vi "Hit Splitter.vi"(8 "error in (no error)":errorcluster, 10 "Coords":T2, 11 "IContainer in":refnum<class "IContainer.lvclass">) -> (0 "error out":errorcluster, 1 "Hit?":bool, 2 "Limits":cluster{"Left":i16, "Right":i16}, 3 "IContainer out":refnum<class "IContainer.lvclass">, 4 "Slider":T1={"Left"=0.0, "Top"=0.0, "Right"=1.0, "Bottom"=0.0}, 5 "vertical?":bool, 6 "Position":i16)   [LabVIEW 2021, in "IContainer.lvclass"]
doc: "Copyright 2018, Wiebe Walstra, wiebe@carya.nl."
uses:
  IContainer.lvclass
  <vilib>/Utility/miscctls.llb/LVPoint32TypeDef.ctl
  IContainer.lvclass/IContainer.ctl
  IObject.lvclass
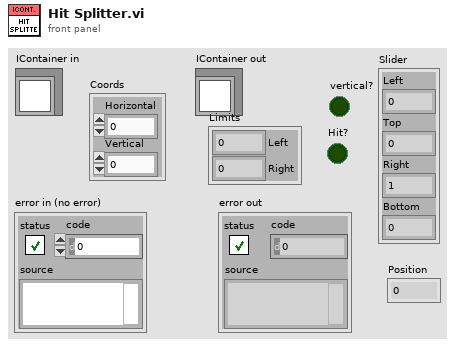
[diagram p1: front panel]
types:
  T1 = cluster{"Left":dbl, "Top":dbl, "Right":dbl, "Bottom":dbl}
  T2 = typedef "LVPoint32TypeDef.ctl" = cluster{"Horizontal":i32, "Vertical":i32}
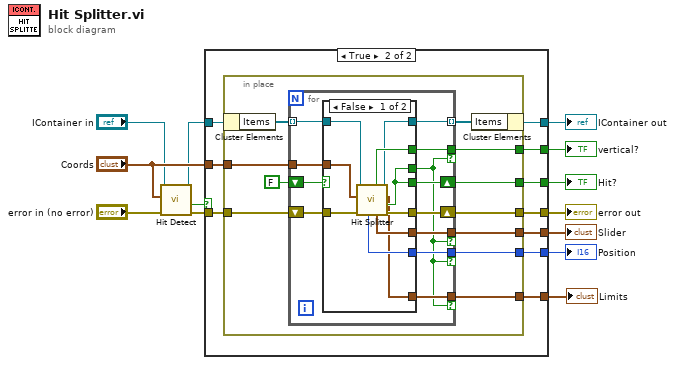
[diagram p0: block diagram]
diagram:
  n1 = call-dynamic "Hit Detect.vi"("error in (no error)"="error in (no error)", "Coords"="Coords", "IContainer in"="IContainer in") -> ("error out"=w8:errorcluster, "Hit?"=w3:bool, "IContainer out"=w1:refnum<class "IContainer.lvclass">)  [unwired: 5 in, 1 out]
  n2 = case shown="True" w3 {
    tunnel: [w15 w25] -> w13
    tunnel: [_ w24] -> w12
    tunnel: [_ w23] -> w11
    tunnel: [_ w22] -> w9
    tunnel: w8 -> [w15 w21]
    tunnel: w1 -> [w14 w18]
    tunnel: "Coords" -> [_ w20]
    tunnel: [w14 w17] -> w7
    tunnel: [_ w19] -> w6
    tunnel: [_ w16] -> w5
    frame False {
    }
    frame True {
      n3 = in-place {
        in-place-border: [w36] -> w25
        in-place-border: [w35] -> w24
        in-place-border: [w34] -> w23
        in-place-border: [w33] -> w22
        in-place-border: w21 -> [w32]
        in-place-border: w20 -> [w31]
        in-place-border: [w30] -> w19
        in-place-border: [w26] -> w16
        n4 = in-place-cluster #1(w18) -> ("Items"=w29:refnum<class "IObject.lvclass">[])
        n5 = for {
          tunnel: [w43] -> w34 if=w37
          tunnel: w31 -> [w46]
          shift-right: [w48] -> w36
          shift-left: w32 -> [w47]
          tunnel: [w45] -> w33 if=w37
          tunnel: [w44] -> w30 if=w37
          tunnel: w29 -> [w42] mode=indexing
          tunnel: [w41] -> w28 mode=indexing
          shift-right: [w39] -> w35
          shift-left: FALSE ("Hit?") -> [w40]
          tunnel: [w38] -> w26 if=w37
          n6 = case shown="False" w40 {
            selector: w40 -> [_ w60]
            tunnel: [w58 w59] -> w48
            tunnel: w47 -> [w57 w59]
            tunnel: w46 -> [w56 _]
            tunnel: [w55 _] -> w45
            tunnel: [w54 _] -> w44
            tunnel: [w53 _] -> w43
            tunnel: w42 -> [w52 w61]
            tunnel: [w51 w61] -> w41
            tunnel: [w50 w60] -> w39
            tunnel: [w50 _] -> w37
            tunnel: [w49 _] -> w38
            frame False {
              n7 = call-dynamic "Hit Splitter.vi"("error in (no error)"=w57, "Point32"=w56, "IObject in"=w52) -> ("error out"=w58:errorcluster, "Hit?"=w50:bool, "Limits"=w49:cluster{"Left":i16, "Right":i16}, "IObject out"=w51:refnum<class "IObject.lvclass">, "Slider"=w53:T1, "vertical?"=w55:bool, "Position"=w54:i16)  [unwired: 2 in]
            }
            frame True {
            }
          }
        }
        n8 = in-place-cluster #1("Items"=w28) -> (w17:refnum<class "IContainer.lvclass">)
      }
    }
  }
  "error out" <- w13
  "IContainer out" <- w7
  "Slider" <- w11
  "Hit?" <- w12
  "vertical?" <- w9
  "Position" <- w6
  "Limits" <- w5
